vi "PH_HamamatsuCamera.PC set Timeout.vi"(0 "i ref in":refnum<vi>, 2 "Timeout":u32, 5 "error in (no error)":errorcluster) -> (14 "i ref out":refnum<vi>, 19 "error out":errorcluster)   [LabVIEW 2014, in "PH_HamamatsuCamera.lvlib"]
doc: "This VI checks whether the incoming value for gain is already applied. If not, it sets the new value to the attributes and the related GUI elements."
uses:
  PH_HamamatsuCamera.lvlib
  PH_Common/PH_Common.lvlib
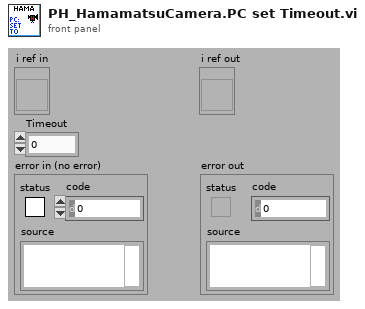
[diagram p1: front panel]
types:
  T1 = typedef "PH_HamamatsuCamera.lvlib/PH_HamamatsuCamera.i attribute.ctl" = cluster{"Gui Refs":cluster{"Camera Details":refnum<vi>, "ROI":refnum<vi>, "Set ROI to Maximum":refnum<vi>, "Trigger Parameters":refnum<vi>, "Brightness":refnum<vi>, "Shutter":refnum<vi>, "Gain":refnum<vi>, "Trigger Timeout":refnum<vi>, "Trigger Polarity":refnum<vi>, "Trigger Mode":refnum<vi>, "Parameters":refnum<vi>, "Set Cam Parameter":refnum<vi>, "Parameter to set":refnum<vi>, "Value to set":refnum<vi>}, "Cam":cluster{"Handle":i32, "Details":cluster{"Model":string, "Camera ID":string, "Firmware":string}, "Buffer Info":cluster{"height":u32, "width":u32, "datatype":u32}}, "H Offset":cluster{"Value":i32, "Minimum":i32, "Maximum":i32, "Increment":i32}, "V Offset":cluster{"Value":i32, "Minimum":i32, "Maximum":i32, "Increment":i32}, "H Width":cluster{"Value":i32, "Minimum":i32, "Maximum":i32, "Increment":i32}, "V Width":cluster{"Value":i32, "Minimum":i32, "Maximum":i32, "Increment":i32}, "Trigger Parameters":T2, "Trigger Timeout":u32, "Parameters":T3[], "Indicees Cam Parameters":cluster{"Brightness":i32, "Shutter":i32, "Gain":i32}, "Wanted Values":cluster{"Trigger Settings":T2[], "ROI":T4[], "Parameter":cluster{"Name":string, "Value":dbl}[]}}
  T2 = typedef "PH_HamamatsuCamera.lvlib/PH_HamamatsuCamera.Trigger Parameter.ctl" = cluster{"Mode":u32, "Polarity":u32, "Times":u32, "Delay":dbl}
  T3 = typedef "PH_HamamatsuCamera.lvlib/PH_HamamatsuCamera.Parameter Set.ctl" = cluster{"Parameter":string, "Value":dbl, "Writable":bool, "Range":cluster{"min":dbl, "max":dbl, "step":dbl}, "Default":dbl, "Value Names":cluster{"Name":string, "Value":dbl}[], "Text Values":bool}
  T4 = typedef "PH_HamamatsuCamera.lvlib/PH_HamamatsuCamera.ROI.ctl" = cluster{"Horizontal Offset":i32, "Vertical Offset":i32, "Horizontal Width":i32, "Vertical Width":i32}
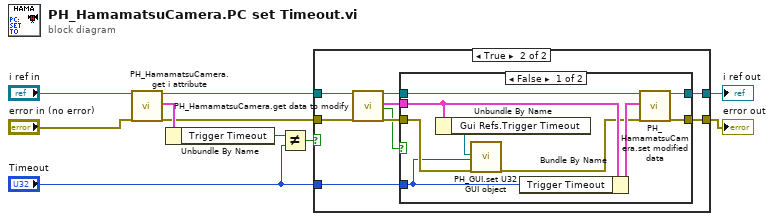
[diagram p0: block diagram]
diagram:
  n1 = call "PH_HamamatsuCamera.get i attribute.vi"("i ref in"="i ref in", "error in (no error)"="error in (no error)") -> ("i ref out"=w7:refnum<vi>, "i attribute"=w10:T1, "error out"=w5:errorcluster)  [unwired: 15 in]
  n2 = Unbundle By Name(w10) -> ("Trigger Timeout"=w2:u32)
  n3 = Not Equal?(x=w2, y="Timeout") -> (x != y?=w3:bool)
  n4 = case shown="True" w3 {
    tunnel: w7 -> [w12 w21]
    tunnel: [w12 w14] -> w6
    tunnel: w5 -> [w11 w20]
    tunnel: [w11 w13] -> w4
    tunnel: "Timeout" -> [_ w16]
    frame False {
    }
    frame True {
      n5 = call "PH_HamamatsuCamera.get data to modify.vi"("i ref in"=w21, "error in (no error)"=w20) -> ("i ref out"=w19:refnum<vi>, "i attribute"=w17:T1, "timed out"=w15:bool, "error out"=w18:errorcluster)  [unwired: 14 in]
      n6 = case shown="False" w15 {
        tunnel: w19 -> [w30 w32]
        tunnel: [w29 w32] -> w14
        tunnel: w18 -> [w25 w31]
        tunnel: [w28 w31] -> w13
        tunnel: w17 -> [w26 _]
        tunnel: w16 -> [w23 _]
        frame False {
          n7 = Unbundle By Name(w26) -> ("Gui Refs.Trigger Timeout"=w22:refnum<vi>)
          n8 = call "PH_GUI.set U32 GUI object.vi"("U32 Ref"=w22, "Value"=w23, "error in (no error)"=w25) -> ("error out"=w24:errorcluster)  [unwired: 16 in]
          n9 = Bundle By Name(cluster=w26, "Trigger Timeout"=w23) -> (w27:T1)
          n10 = call "PH_HamamatsuCamera.set modified data.vi"("i ref in"=w30, "i attribute"=w27, "error in (no error)"=w24) -> ("i ref out"=w29:refnum<vi>, "error out"=w28:errorcluster)  [unwired: 15 in]
        }
        frame True {
        }
      }
    }
  }
  "i ref out" <- w6
  "error out" <- w4
